vi "Publish Values.vi"(8 "error in (no error)":errorcluster, 11 "SoftVar Module in":refnum<class "SoftVar Module.lvclass">) -> (0 "error out":errorcluster, 3 "SoftVar Module out":refnum<class "SoftVar Module.lvclass">)   [LabVIEW 2020, in "Volatus.lvlib" / "SoftVar Module.lvclass"]
uses:
  SoftVar Module.lvclass
  SoftVar Module.lvclass/SoftVar Module.ctl
  Module/Module.lvclass
  C:/dev/lv20CE/relink/lv-volatus/Volatus/Module/Module.lvclass
  C:/dev/lv20CE/relink/lv-volatus/Volatus/SoftVar Module/SoftVar Module.lvclass
  VolatusAPI/VolatusAPI.lvclass
  lv-vecto/Vecto/Group/Group.lvclass
  C:/dev/lv20CE/relink/lv-vecto/Vecto/GroupAbstract/GroupAbstract.lvclass
  C:/dev/lv20CE/relink/lv-vecto/Vecto/Group/Group.lvclass
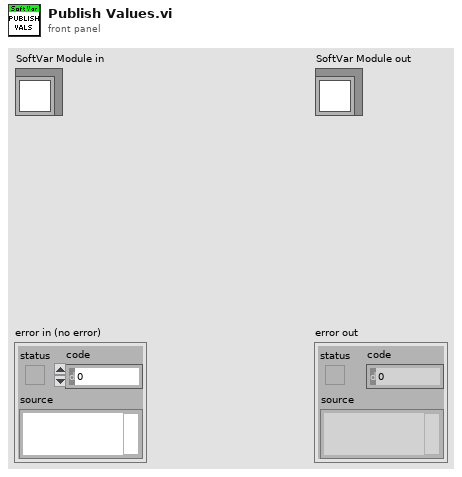
[diagram p1: front panel]
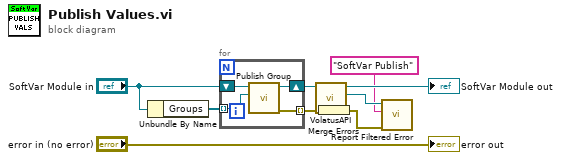
[diagram p0: block diagram]
diagram:
  n1 = Unbundle By Name("SoftVar Module in") -> ("Groups"=w6:refnum<class "Group.lvclass">[])
  n2 = for {
    shift-right: [w12] -> w7
    shift-left: "SoftVar Module in" -> [w13]
    tunnel: w6 -> [w11] mode=indexing
    tunnel: [w10] -> w4 mode=indexing
    n3 = call "Publish Group.vi"("Group"=w11, "Module in"=w13) -> ("error out"=w10:errorcluster, "Module out"=w12:refnum<class "SoftVar Module.lvclass">)  [unwired: 8 in]
  }
  n4 = call "VolatusAPI.vi"("Module in"=w7) -> ("VolatusAPI"=w2:refnum<class "VolatusAPI.lvclass">, "Module out"=→"SoftVar Module out":refnum<class "SoftVar Module.lvclass">)  [unwired: 9 in]
  n5 = Merge Errors(w4) -> (w3:errorcluster)
  n6 = call "Report Filtered Error.vi"("error in (no error)"=w3, "Context"="SoftVar Publish", "VolatusAPI in"=w2) -> ()  [unwired: 7 in, 2 out]
  "error out" <- "error in (no error)"
